vi "SistemaCalentadorAgua.vi"() -> ()   [LabVIEW 2010]
uses:
  <vilib>/Platform/TimedLoop/XDataNode/XDataNode.xnode
  <vilib>/Platform/TimedLoop/XDataNode/timing_clust.ctl
  <vilib>/Platform/TimedLoop/XDataNode/nitl_modes.ctl
  <vilib>/Platform/TimedLoop/XDataNode/wakeup.ctl
  <vilib>/Instr/_visa.llb/VISA Configure Serial Port (Instr).vi
  <vilib>/Platform/TimedLoop/XDataNode/XDNodeRunTimeDep.lvlib
panel:
  out "Posicion Real Esfera (mm)":dbl(slide) scale=10.0..60.0
  in  "Ajuste":i16(slide) scale=0.0..10.0
  out "Temperatura actual vs t":dynamicdata(graph)
  in  "Set Posicion":i16(slide) scale=0.0..60.0
  out "?":bool
  in  "Period                :":i64=1000
  in  "Flow control    :":u16(ring) items=["None"=0, "XON/XOFF"=1, "RTS/CTS"=2, "DTR/DSR"=4]
  in  "Stop bits         :":u16(ring)=10 items=["1.0"=10, "1.5"=15, "2.0"=20]
  in  "Paridad            :":u16(ring) items=["None", "Odd", "Even", "Mark", "Space"]
  in  "Data bits          :":u16=8 min=5 max=8 step=1
  in  "VISA resource : name:":refnum<visa-resource-name>="COM1"
  in  "Baud rate         :":u32=9600
  in  "stop":bool
  out "Read buffer":string
  out "var p":i32
  # "Sistema de equilibrio de una esfera"
  # "Configuracion Serial"
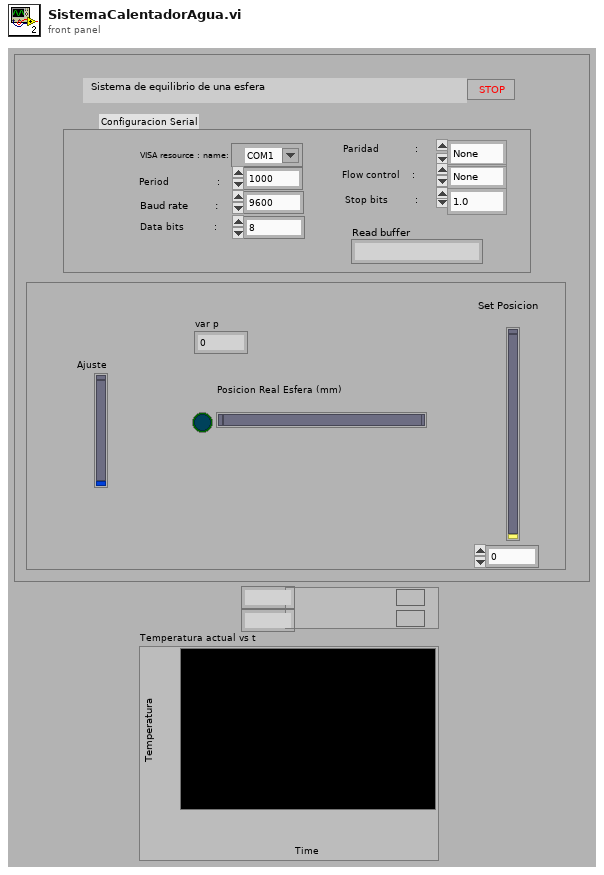
[diagram p1: front panel]
types:
  T1 = typedef "XDNodeRunTimeDep.lvlib/timing_clust.ctl" = cluster{"Expected End [f-1]":u64, "Actual End [f-1]":u64, "Finished Late? [f-1]":bool, "Expected End [i-1]":u64, "Actual End [i-1]":u64, "Finished Late? [i-1]":bool, "Expected Start [i]":u64, "Actual Start [i]":u64, "Expected Start [f]":u64, "Actual Start [f]":u64, "Source Name":string, "Structure Name":string, "Period":i64, "Deadline":i64, "Offset":i64, "Start":i64, "Priority":i32, "Timeout":i32, "Mode":T2, "Wakeup Reason":T3, "Error":errorcluster, "Source Type":string, "Secondary Source Type":string, "Global End Time":u64, "Global Start Time":u64, "Frame Duration":u64, "Iteration Duration":u64, "Assigned CPU":i32, "I/O Scan Engine Mode":u32}
  T2 = typedef "XDNodeRunTimeDep.lvlib/nitl_modes.ctl" = enum32{"No Change", "Process missed periods, maintain original phase", "Discard missed periods, maintain original phase", "Process missed periods, ignore original phase", "Discard missed periods, ignore original phase"}
  T3 = typedef "XDNodeRunTimeDep.lvlib/wakeup.ctl" = enum32{"Normal", "Aborted", "Asynchronous wakeup", "Timing source error", "Timed loop error", "Timeout"}
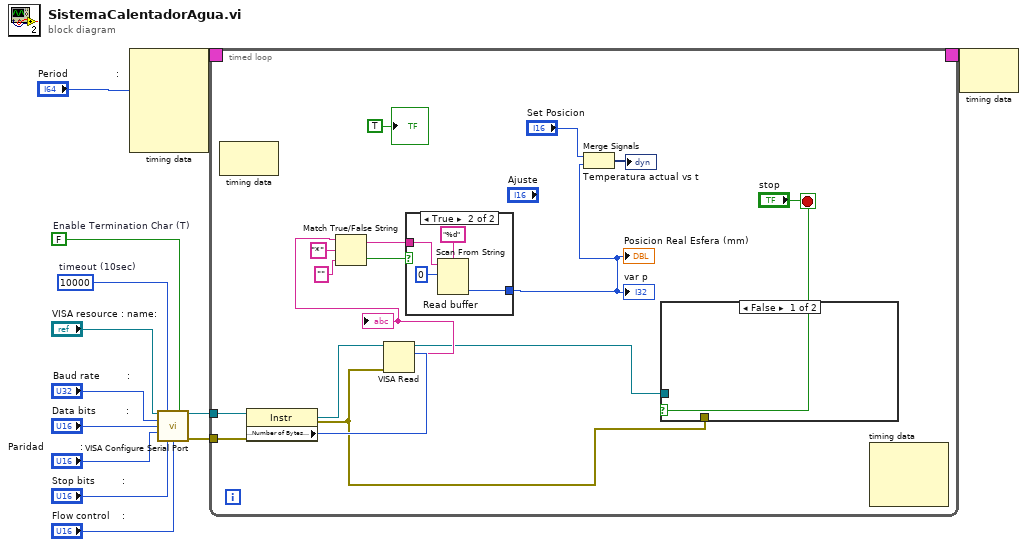
[diagram p0: block diagram]
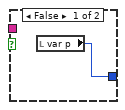
[diagram p2: hidden frame]
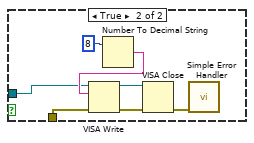
[diagram p3: hidden frame]
diagram:
  w7 = FALSE  # Enable Termination Char (T)
  w8 = u32 10000  # timeout (10sec)
  n1 = node-c288("Period                :") -> (w13:T1)  [unwired: 4 in]
  n2 = call-poly "VISA Configure Serial Port"("VISA resource name"="VISA resource : name:", "timeout (10sec)"=w8, "Enable Termination\nChar (T)"=w7, "baud rate (9600)"="Baud rate         :", "data bits (8)"="Data bits          :", "parity (0:none)"="Paridad            :", "stop bits (10: 1 bit)"="Stop bits         :", "flow control (0:none)"="Flow control    :") -> ("VISA resource name out"=w3:refnum<visa-resource-name>, "error out"=w2:errorcluster)  [unwired: 6 in]
  n3 = timed-loop {
    timing: w13 -> [_]
    timing-out: [_] -> w12
    tunnel: w3 -> [w26]
    tunnel: w2 -> [w25]
    stop <- "stop" stop-if-true
    n4 = node-c288() -> ()  [unwired: 1 in, 1 out]
    n5 = property class="Instr"(reference=w26, error in=w25) -> (reference out=w27:refnum<visa-resource-name>, error out=w24:errorcluster, "Serial Settings:Number of Bytes at Serial Port"=w29:u32)
    n6 = VISA Read(VISA resource name=w27, byte count=w29, error in (no error)=w24) -> (VISA resource name out=w17:refnum<visa-resource-name>, read buffer=w18:string)  [unwired: 2 out]
    "Read buffer" <- w18
    n7 = Match True/False String(2:"" ("false string"), 3:"*" ("true string"), 4:w18) -> (0:w20:bool, 1:w19:string)
    n8 = case shown="True" w20 {
      tunnel: [w30 w32] -> w14
      tunnel: w19 -> [_ w31]
      frame False {
        n9 = local read "var p"() -> (w30:i32)
      }
      frame True {
        n10 = Scan From String(format string="%d", input string=w31, initial scan location=u32 0) -> (output 1=w32:i32)  [unwired: 2 in, 3 out]
      }
    }
    "var p" <- w14
    "Posicion Real Esfera (mm)" <- w14
    n11 = Merge Signals("Set Posicion", w14) -> (→"Temperatura actual vs t":dynamicdata)
    n12 = case shown="False" "stop" {
      tunnel: w17 -> [_ w36]
      tunnel: w24 -> [_ w35]
      frame False {
      }
      frame True {
        n13 = Number To Decimal String(number=8) -> (decimal integer string=w37:string)  [unwired: 1 in]
        n14 = VISA Write(VISA resource name=w36, write buffer=w37, error in (no error)=w35) -> (VISA resource name out=w39:refnum<visa-resource-name>, error out=w38:errorcluster)  [unwired: 1 out]
        n15 = VISA Close(VISA resource name=w39, error in (no error)=w38) -> (error out=w41:errorcluster)
        n16 = call <vilib>:"Simple Error Handler.vi"("error in (no error)"=w41) -> ()  [unwired: 4 in, 5 out]
      }
    }
    n17 = node-c288() -> ()  [unwired: 3 in, 1 out]
    "?" <- TRUE
  }
  n18 = node-c288(w12) -> ()  [unwired: 1 out]
